vi "Start Chroma.vi"(4 "ReadTimeout(10000)":u32=12000, 6 "Port Timeout":u32=500, 8 "ErrOut":errorcluster, 11 "VISA resource name":refnum<visa-resource-name>="com21") -> (0 "ErrOutResult?":errorcluster, 1 "ReadResultErr":bool caption="讀取錯誤", 2 "Ary_CurrentReadOut":dbl[](array[numeric]), 3 "OK":bool[](array[boolean]), 5 "send":string[](array[string]), 7 "reply":string[](array[string]))   [LabVIEW 2016]
uses:
  DISGradingMachine/global value.vi
  <vilib>/Instr/_visa.llb/VISA Configure Serial Port (Instr).vi
panel:
  out "Array 2":T1(array[ring])
  out "ErrOutStart":errorcluster
  # "TV量測中,請稍候........."
  # "升壓中,高壓危險 請勿觸碰測座"
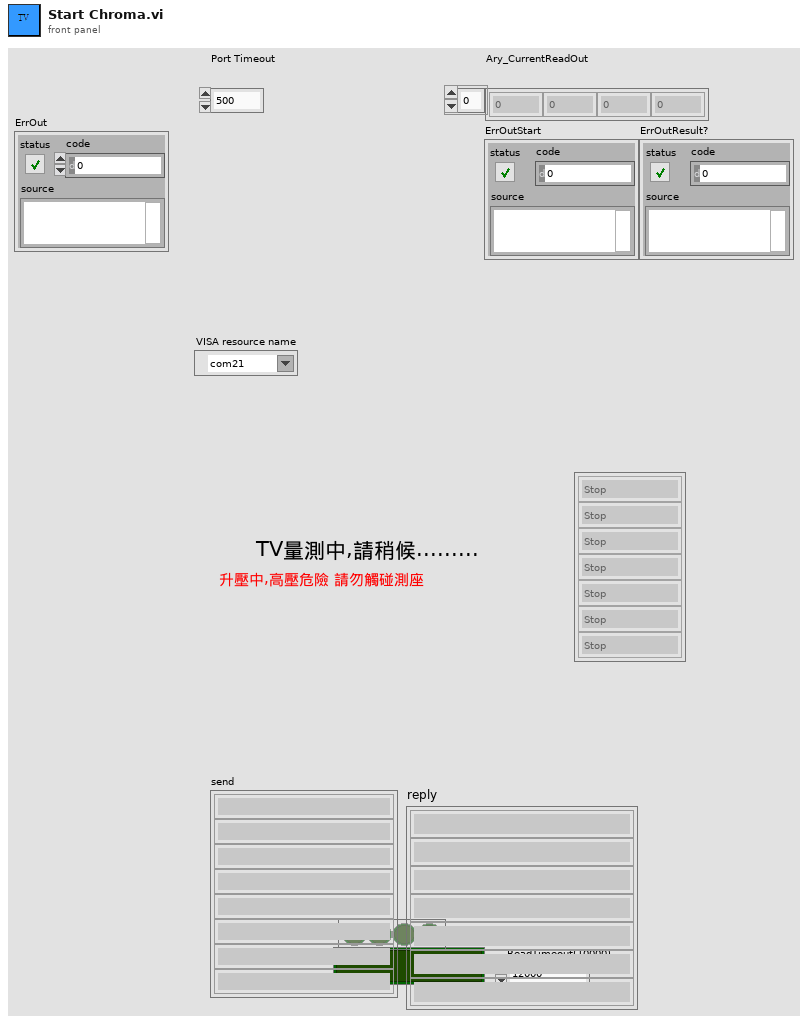
[diagram p1: front panel]
types:
  T1 = enum8{"Stop", "User Interupt", "Can not test", "Testing", "Pass", "Skipped", "GFI Tripped"}[]
  T2 = enum16{"IDN?", "test", "Stop", "Start", "Step Parameters", "Step Patameters?", "Preset Parameter", "Preset parameter?", "Offset Get/Off", "Offset?", "System Setting", "System Setting?", "KeyLock", "KeyLock?", "Initialize All Steps Parameter", "Remote/Local", "Result"}
  T3 = cluster{"EnumFunnction":enum16{"IDN?", "test", "Stop", "Start", "Step Parameters", "Step Patameters?", "Preset Parameter", "Preset parameter?", "Offset Get/Off", "Offset?", "System Setting", "System Setting?", "KeyLock", "KeyLock?", "Initialize All Steps Parameter", "Remote/Local", "Result"}, "Hex_DA":u8, "Hex_Master":u8}
  T4 = enum8{"Stop", "User Interupt", "Can not test", "Testing", "Pass", "Skipped", "GFI Tripped"}
  T5 = cluster{"Mode":enum8{"Non", "AC", "DC", "IR"}, "Meter1(Source)":u16, "Meter2(Current,Resistance)":u32, "Meter3(Inrush)":u32, "RampTime":u16, "DwellTime":u16, "Testtime":u16, "FallTime":u16, "BooleanFlag":bool, "int_step":u8, "Enum_ResultType":enum8{"Stop", "User Interupt", "Can not test", "Testing", "Pass", "Skipped", "GFI Tripped"}}
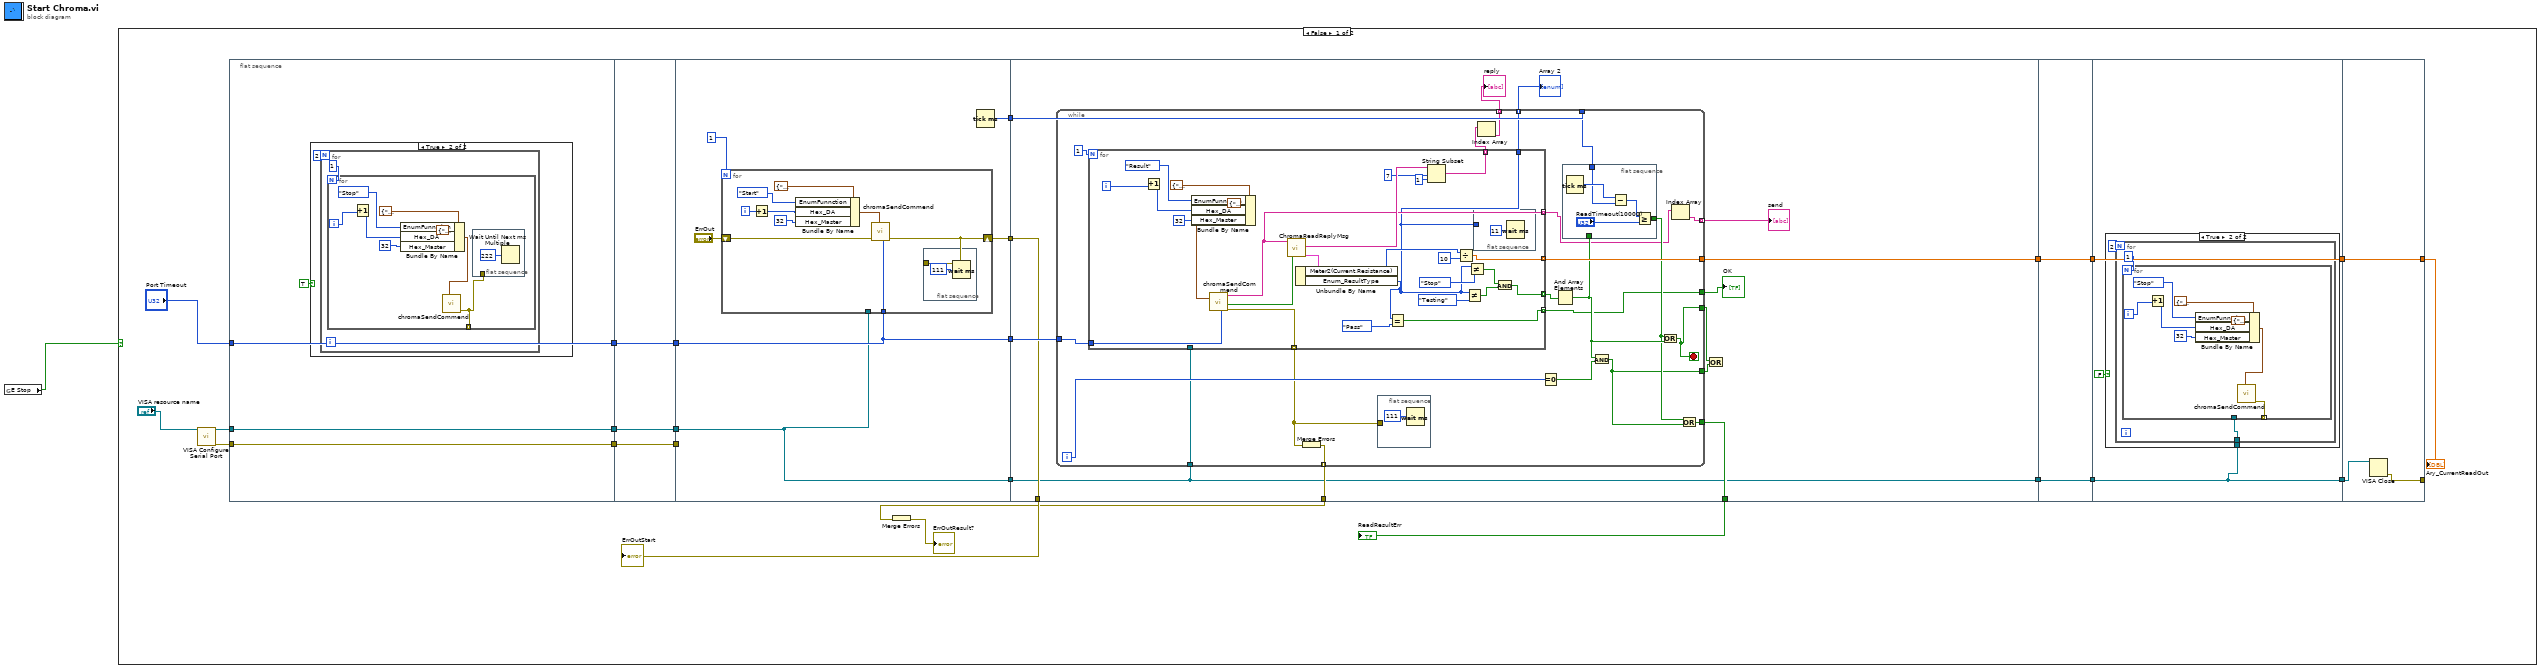
[diagram p0: block diagram]
diagram:
  n1 = global read "global value.vi" "E Stop"() -> (w1:bool)
  n2 = case shown="False" w1 {
    frame False {
      n3 = call-poly "VISA Configure Serial Port"("VISA resource name"="VISA resource name") -> ("VISA resource name out"=w14:refnum<visa-resource-name>, "error out"=w17:errorcluster)  [unwired: 13 in]
      n4 = flat-sequence {
        tunnel: w14 -> [w28]
        tunnel: w17 -> [w29]
        tunnel: "Port Timeout" -> [w30]
        tunnel: [w30] -> w7
        tunnel: [w29] -> w5
        tunnel: [w28] -> w3
        tunnel: w7 -> [w43]
        tunnel: [w43] -> w6
        tunnel: w5 -> [w42]
        tunnel: [w42] -> w4
        tunnel: w3 -> [w41]
        tunnel: [w41] -> w2
        tunnel: [w47] -> w26
        tunnel: [w46] -> w25
        tunnel: [w45] -> w24
        tunnel: [w44] -> w15
        tunnel: w6 -> [w47]
        tunnel: w4 -> [_]
        tunnel: w2 -> [w44]
        tunnel: w26 -> [w72]
        tunnel: w25 -> [w71]
        tunnel: w24 -> [w69]
        tunnel: [w69] -> w21
        tunnel: [w68] -> w20
        tunnel: [w65] -> w18
        tunnel: [w70] -> w11
        tunnel: w15 -> [w63]
        tunnel: [w63] -> w9
        tunnel: w11 -> [w128]
        tunnel: [w128] -> w10
        tunnel: w9 -> [w127]
        tunnel: [w127] -> w8
        tunnel: w10 -> [w131]
        tunnel: [w131] -> w13
        tunnel: w8 -> [w129]
        tunnel: [w129] -> w12
        tunnel: [w145] -> w22
        tunnel: w13 -> [w145]
        tunnel: [w144] -> _
        tunnel: w12 -> [w143]
        frame #0 {
          n5 = case shown="True" TRUE {
            frame False {
            }
            frame True {
              n6 = for {
                N: 2 -> [_]
                n7 = for {
                  N: 1 -> [_]
                  tunnel: [w33] -> _ mode=indexing
                  i -> [w35]
                  (unwired) T3 {"EnumFunnction"=enum."Preset Parameter", "Hex_DA"=1, "Hex_Master"=32} ("Clus_STDparameter")
                  n8 = Increment(x=w35) -> (x+1=w38:i32)
                  n9 = Bundle By Name(cluster=T3 {"EnumFunnction"=enum."Preset Parameter", "Hex_DA"=1, "Hex_Master"=32} ("Clus_STDparameter"), "EnumFunnction"=T2."Stop", "Hex_DA"=w38, "Hex_Master"=u8 32) -> (w34:T3)
                  n10 = call "chromaSendCommend.vi"("Clus_STDparameter"=w34) -> ("ErrOut"=w33:errorcluster)  [unwired: 7 in, 3 out]
                  n11 = flat-sequence {
                    tunnel: w33 -> [_]
                    frame #0 {
                      n12 = Wait Until Next ms Multiple(millisecond multiple=u32 222) -> ()  [unwired: 1 out]
                    }
                  }
                }
              }
            }
          }
        }
        frame #1 {
        }
        frame #2 {
          n13 = for {
            N: 1 -> [_]
            shift-right: [w51] -> w45
            shift-left: "ErrOut" -> [w57]
            tunnel: w47 -> [w50]
            tunnel: w44 -> [_]
            i -> [w58]
            n14 = Increment(x=w58) -> (x+1=w54:i32)
            n15 = Bundle By Name(cluster=T3 {"EnumFunnction"=enum."Preset Parameter", "Hex_DA"=1, "Hex_Master"=32} ("Clus_STDparameter"), "EnumFunnction"=T2."Start", "Hex_DA"=w54, "Hex_Master"=u8 32) -> (w56:T3)
            n16 = call "chromaSendCommend.vi"("Int_Port Timeout"=w50, "Clus_STDparameter"=w56, "ErrIn"=w57) -> ("ErrOut"=w51:errorcluster)  [unwired: 5 in, 3 out]
            n17 = flat-sequence {
              tunnel: w51 -> [_]
              frame #0 {
                n18 = Wait (ms)(milliseconds to wait=u32 111) -> ()  [unwired: 1 out]
              }
            }
          }
          n19 = Tick Count (ms)() -> (millisecond timer value=w46:u32)
        }
        frame #3 {
          n20 = while {
            tunnel: w72 -> [w92]
            tunnel: w71 -> [w90]
            tunnel: [w89] -> w70
            tunnel: [w82] -> w67
            tunnel: [w85] -> w68 mode=indexing
            tunnel: [w84] -> w66
            tunnel: [w81] -> w65
            tunnel: [w80] -> w64
            tunnel: w63 -> [w78]
            tunnel: [w76] -> w62 mode=indexing
            tunnel: [w74] -> w61 mode=indexing
            tunnel: [w73] -> w60 mode=indexing
            i -> [w88]
            stop <- w84 stop-if-true
            n21 = for {
              N: 1 -> [_]
              tunnel: w92 -> [w119]
              tunnel: [w100] -> w91 mode=indexing
              tunnel: [w115] -> w89 mode=indexing
              tunnel: [w114] -> w79 mode=indexing
              tunnel: [w111] -> w80 mode=indexing
              tunnel: [w107] -> w77 mode=indexing
              tunnel: [w103] -> w73
              tunnel: w78 -> [_]
              tunnel: [w105] -> w75 mode=indexing
              i -> [w121]
              (unwired) T3 {"EnumFunnction"=enum."Preset Parameter", "Hex_DA"=1, "Hex_Master"=32} ("Clus_STDparameter")
              n22 = Increment(x=w121) -> (x+1=w124:i32)
              n23 = Bundle By Name(cluster=T3 {"EnumFunnction"=enum."Preset Parameter", "Hex_DA"=1, "Hex_Master"=32} ("Clus_STDparameter"), "EnumFunnction"=T2."Result", "Hex_DA"=w124, "Hex_Master"=u8 32) -> (w120:T3)
              n24 = call "chromaSendCommend.vi"("Int_Port Timeout"=w119, "Clus_STDparameter"=w120) -> ("ErrOut"=w114:errorcluster, "ChecksumError"=w113:bool, "Str_ ReplyStr"=w105:string)  [unwired: 6 in, 1 out]
              n25 = call "ChromaReadReplyMsg.vi"("Boolean_MsgReceiveErr?"=w113, "Str_ReplyIn"=w105) -> ("Clu_Result?"=w106:T5, "Str_MsgOut"=w110:string)  [unwired: 3 in, 5 out]
              n26 = Unbundle By Name(w106) -> ("Meter2(Current,Resistance)"=w117:u32, "Enum_ResultType"=w103:T4)
              n27 = Equal?(x=w103, y=T4."Pass" ("Enum_ResultType")) -> (x = y?=w111:bool)
              n28 = String Subset(string=w110, offset (0)=7, length (rest)=1 ("length (rest)")) -> (substring=w107:string)
              n29 = Divide(x=w117, y=u16 10) -> (x/y=w115:dbl)
              n30 = Not Equal?(x=w103, y=T4."Testing" ("Enum_ResultType")) -> (x != y?=w101:bool)
              n31 = Not Equal?(x=w103, y=T4."Stop" ("Enum_ResultType")) -> (x != y?=w102:bool)
              n32 = flat-sequence {
                tunnel: w103 -> [_]
                frame #0 {
                  n33 = Wait (ms)(milliseconds to wait=u32 11) -> ()  [unwired: 1 out]
                }
              }
              n34 = And(x=w102, y=w101) -> (x .and. y?=w100:bool)
            }
            n35 = Merge Errors(w79) -> (w85:errorcluster)
            n36 = flat-sequence {
              tunnel: w79 -> [_]
              frame #0 {
                n37 = Wait (ms)(milliseconds to wait=u32 111) -> ()  [unwired: 1 out]
              }
            }
            n38 = Index Array(array=w77) -> (element=w76:string)  [unwired: 1 in]
            n39 = Equal To 0?(x=w88) -> (x = 0?=w86:bool)
            n40 = And Array Elements(Boolean array=w91) -> (logical AND=w87:bool)
            n41 = flat-sequence {
              tunnel: w90 -> [w98]
              tunnel: w87 -> [_]
              tunnel: [w95] -> w83
              frame #0 {
                n42 = Tick Count (ms)() -> (millisecond timer value=w99:u32)
                n43 = Subtract(x=w99, y=w98) -> (x-y=w97:u32)
                n44 = Greater Or Equal?(x=w97, y="ReadTimeout(10000)") -> (x >= y?=w95:bool)
              }
            }
            n45 = And(x=w87, y=w86) -> (x .and. y?=w82:bool)
            n46 = Or(x=w83, y=w87) -> (x .or. y?=w84:bool)
            n47 = Index Array(array=w75) -> (element=w74:string)  [unwired: 1 in]
            n48 = Or(x=w83, y=w82) -> (x .or. y?=w81:bool)
          }
          "OK" <- w64
          "reply" <- w62
          "send" <- w61
          "Array 2" <- w60
          n49 = Or(x=w66, y=w67) -> ()  [unwired: 1 out]
        }
        frame #4 {
        }
        frame #5 {
          n50 = case shown="True" FALSE {
            tunnel: w129 -> [_ w133]
            frame False {
            }
            frame True {
              n51 = for {
                N: 2 -> [_]
                tunnel: w133 -> [w134]
                n52 = for {
                  N: 1 -> [_]
                  tunnel: [w136] -> _ mode=indexing
                  tunnel: w134 -> [_]
                  i -> [w138]
                  (unwired) T3 {"EnumFunnction"=enum."Preset Parameter", "Hex_DA"=1, "Hex_Master"=32} ("Clus_STDparameter")
                  n53 = Increment(x=w138) -> (x+1=w141:i32)
                  n54 = Bundle By Name(cluster=T3 {"EnumFunnction"=enum."Preset Parameter", "Hex_DA"=1, "Hex_Master"=32} ("Clus_STDparameter"), "EnumFunnction"=T2."Stop", "Hex_DA"=w141, "Hex_Master"=u8 32) -> (w137:T3)
                  n55 = call "chromaSendCommend.vi"("Clus_STDparameter"=w137) -> ("ErrOut"=w136:errorcluster)  [unwired: 7 in, 3 out]
                }
              }
            }
          }
        }
        frame #6 {
          n56 = VISA Close(VISA resource name=w143) -> (error out=w144:errorcluster)  [unwired: 1 in]
        }
      }
      n57 = Merge Errors(w20) -> (→"ErrOutResult?":errorcluster)
      "Ary_CurrentReadOut" <- w22
      "ErrOutStart" <- w21
      "ReadResultErr" <- w18
    }
    frame True {
    }
  }
